vi "3654AngleDif.vi"(9 "CapturedAngle":dbl, 11 "NewAngle":dbl) -> (3 "AngleDifference":dbl, 8 "Error":dbl)   [LabVIEW 2017]
uses:
  <vilib>/Analysis/coordinate.llb/Angle Range (Degree).ctl
  <vilib>/Analysis/coordinate.llb/Angle Units.ctl
  <vilib>/Analysis/coordinate.llb/Wrap Angle (scalar).vi
  <vilib>/Analysis/NI_AAL_Angle.lvlib
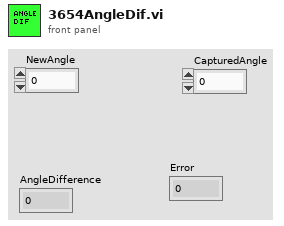
[diagram p1: front panel]
types:
  T1 = typedef "NI_AAL_Angle.lvlib/Angle Units.ctl" = i32
  T2 = typedef "NI_AAL_Angle.lvlib/Angle Range (Degree).ctl" = u16
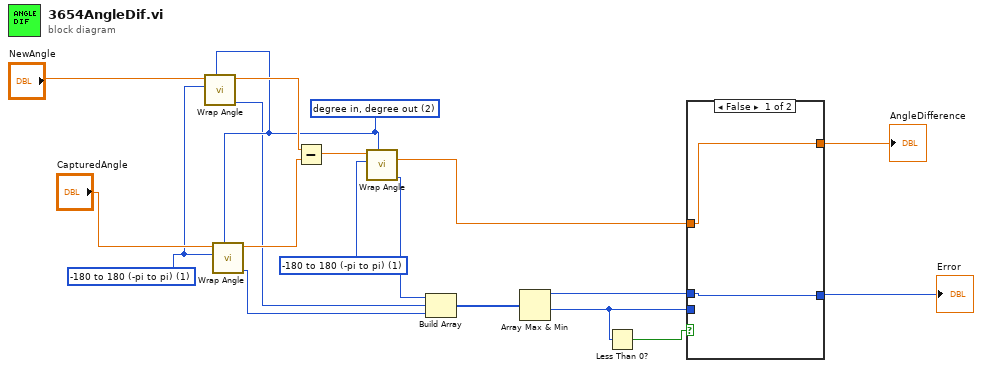
[diagram p0: block diagram]
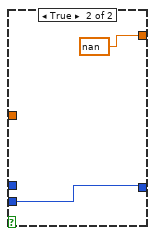
[diagram p2: hidden frame]
diagram:
  w10 = T1 2 items=["radian in, radian out", "radian in, degree out", "degree in, degree out", "degree in, radian out"] ("angle units")
  w11 = T2 1 items=["none", "-180 to 180 (-pi to pi)", "0 to 360 (0 to 2pi)"] ("angle range")
  w12 = T2 1 items=["none", "-180 to 180 (-pi to pi)", "0 to 360 (0 to 2pi)"] ("angle range")
  n1 = call-poly <vilib>:"Wrap Angle.vi"("angle units"=w10, "angle range"=w12, "angle in"="NewAngle") -> ("error"=w8:i32, "angle out"=w15:dbl)  [unwired: 7 in]
  n2 = call-poly <vilib>:"Wrap Angle.vi"("angle units"=w10, "angle range"=w12, "angle in"="CapturedAngle") -> ("error"=w9:i32, "angle out"=w17:dbl)  [unwired: 7 in]
  n3 = Subtract(x=w15, y=w17) -> (x-y=w14:dbl)
  n4 = call-poly <vilib>:"Wrap Angle.vi"("angle units"=w10, "angle range"=w11, "angle in"=w14) -> ("error"=w7:i32, "angle out"=w13:dbl)  [unwired: 7 in]
  n5 = Build Array(w7, w8, w9) -> (w6:i32[])
  n6 = Array Max & Min(array=w6) -> (max value=w5:i32, min value=w3:i32)  [unwired: 2 out]
  n7 = Less Than 0?(x=w3) -> (x < 0?=w4:bool)
  n8 = case shown="False" w4 {
    tunnel: w13 -> [w20 _]
    tunnel: w5 -> [w19 _]
    tunnel: w3 -> [_ w22]
    tunnel: [w19 w22] -> w2
    tunnel: [w20 nan ("AngleDifference")] -> w1
    frame False {
    }
    frame True {
    }
  }
  "AngleDifference" <- w1
  "Error" <- w2
